vi "Tab_In_Out.vi"(10 "Shift?":bool, 11 "String in":refnum<vi>) -> (3 "result string":string)   [LabVIEW 2021]
uses:
  <vilib>/Utility/miscctls.llb/LVSelectionTypeDef.ctl
panel:
  out "x+y":T1
  out "Value 2":string
  out "Text.Selection in":T1
  out "Value":string
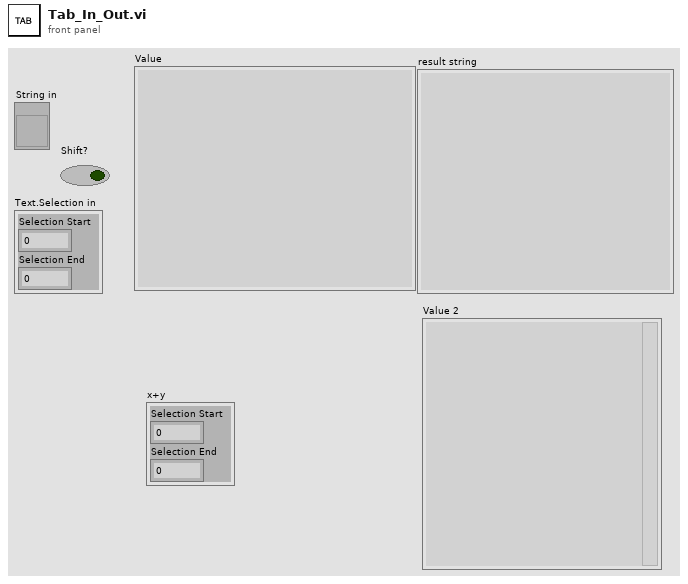
[diagram p1: front panel]
types:
  T1 = typedef "LVSelectionTypeDef.ctl" = cluster{"Selection Start":u32, "Selection End":u32}
  T2 = cluster{"Selection Start":dbl, "Selection End":dbl}
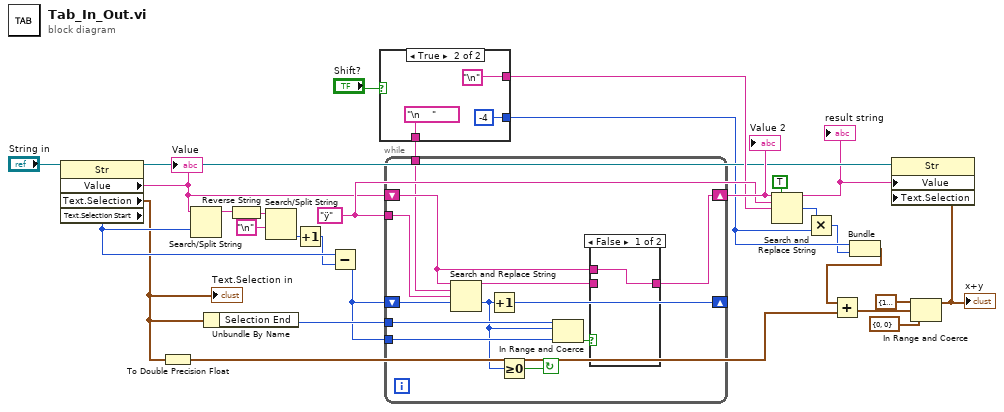
[diagram p0: block diagram]
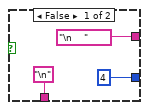
[diagram p2: hidden frame]
diagram:
  w25 = "ÿ" ("replace string (\"\")")
  n1 = property on="Property Node" class="Str"(reference="String in") -> (reference out=w11:refnum<vi>, "Value"=w23:string, "Text.Selection"=w12:T1, "Text.Selection Start"=w19:u32)  [unwired: 1 in, 1 out]
  "Value" <- w23
  "Text.Selection in" <- w12
  n2 = To Double Precision Float(number=w12) -> (double precision float=w7:T2)
  n3 = Search/Split String(string=w23, offset (0)=w19) -> (substring before match=w22:string)  [unwired: 1 in, 2 out]
  n4 = Unbundle By Name(w12) -> ("Selection End"=w27:u32)
  n5 = Reverse String(1:w22) -> (0:w21:string)
  n6 = Search/Split String(string=w21, search string/char (-)="\n") -> (offset of match=w18:i32)  [unwired: 1 in, 2 out]
  n7 = Increment(x=w18) -> (x+1=w17:i32)
  n8 = Subtract(x=w19, y=w17) -> (x-y=w16:u32)
  n9 = case shown="True" "Shift?" {
    tunnel: ["\n" ("regular expression") "\n    " ("regular expression")] -> w14
    tunnel: ["\n    " ("regular expression") "\n" ("regular expression")] -> w13
    tunnel: [4 -4] -> w2
    frame False {
    }
    frame True {
    }
  }
  n10 = while {
    shift-right: [w45] -> _
    shift-left: w16 -> [w46]
    tunnel: w27 -> [w44]
    tunnel: w16 -> [w43]
    shift-right: [w40] -> w26
    shift-left: w23 -> [w38]
    tunnel: w25 -> [w37]
    tunnel: w14 -> [w35]
    stop <- w42 continue-if-true
    n11 = Search and Replace String(input string=w38, search string=w35, replace string=w37, offset=w46) -> (result string=w39:string, offset past replacement=w36:i32)  [unwired: 4 in, 2 out]
    n12 = Increment(x=w36) -> (x+1=w45:i32)
    n13 = Greater Or Equal To 0?(x=w36) -> (x >= 0?=w42:bool)
    n14 = In Range and Coerce(upper limit=w44, x=w36, lower limit=w43) -> (In Range?=w41:bool)  [unwired: 1 out]
    n15 = case shown="False" w41 {
      tunnel: [w47 w48] -> w40
      tunnel: w39 -> [_ w48]
      tunnel: w38 -> [w47 _]
      frame False {
      }
      frame True {
      }
    }
  }
  "Value 2" <- w26
  n16 = Search and Replace String(replace all?=TRUE ("replace all? (F)"), input string=w26, search string=w25, replace string=w13) -> (result string=w10:string, number of replacements=w3:i32)  [unwired: 4 in, 2 out]
  "result string" <- w10
  n17 = Multiply(x=w3, y=w2) -> (x*y=w1:i32)
  n18 = Bundle(w2, w1) -> (w6:cluster{i32, i32})  [unwired: 1 in]
  n19 = Add(x=w6, y=w7) -> (x+y=w5:cluster{dbl, dbl})
  n20 = In Range and Coerce(upper limit=cluster{i32, i32} {100000, 100000}, x=w5, lower limit=cluster{i32, i32} {0, 0}) -> (coerced(x)=w4:cluster{dbl, dbl})  [unwired: 1 out]
  "x+y" <- w4
  n21 = property on="Property Node" class="Str"(reference=w11, "Value"=w10, "Text.Selection"=w4) -> ()  [unwired: 1 in, 2 out]
